vi "move manipulator abs xy.vi"(5 "blocking?":bool=TRUE, 7 "which manipulator":T1(ring), 8 "error in (no error)":errorcluster, 9 "transform cluster + actuator":T2, 10 "positions":T3, 11 "location (steps)":dbl[](array[numeric])) -> (0 "error out":errorcluster)   [LabVIEW 2015]
uses:
  pipette cleaning/pressure box/cleaning_soft/controls/actuator_type.ctl
  pipette cleaning/pressure box/cleaning_soft/controls/actuator_cluster.ctl
  machine_vision/coordinate model vis/transform_properties_actuators.ctl
  machine_vision/controls/transform_cluster_actuator.ctl
panel:
  # "move manip top lvl"
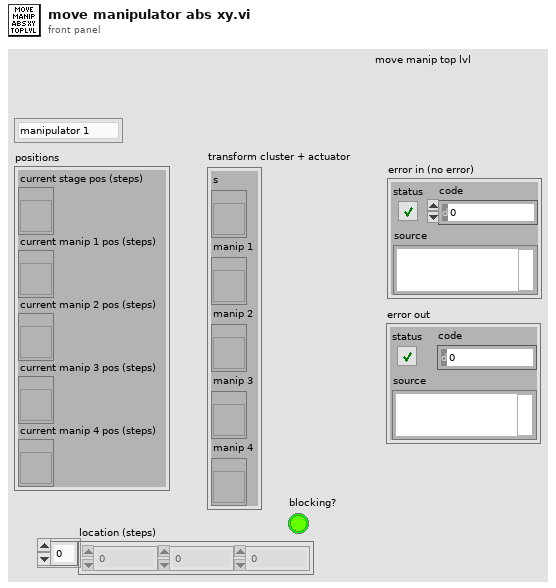
[diagram p1: front panel]
types:
  T1 = enum16{"manipulator 1", "manipulator 2", "manipulator 3", "manipulator 4"}
  T2 = typedef "transform_cluster_actuator.ctl" = cluster{"s":refnum<vi>, "manip 1":refnum<vi>, "manip 2":refnum<vi>, "manip 3":refnum<vi>, "manip 4":refnum<vi>}
  T3 = cluster{"current stage pos (steps)":refnum<vi>, "current manip 1 pos (steps)":refnum<vi>, "current manip 2 pos (steps)":refnum<vi>, "current manip 3 pos (steps)":refnum<vi>, "current manip 4 pos (steps)":refnum<vi>}
  T4 = typedef "transform_properties_actuators.ctl" = cluster{"theta (deg)":dbl, "X sc factor (px/step)":dbl, "Y sc factor (px/step)":dbl, "zero loc (x,y,z)":dbl[], "flip y?":bool, "flip x?":bool, "gamma (deg)":dbl, "flip z?":bool, "Z sc factor (px/step)":dbl, "actuator":T5, "safe space (steps)":i32[]}
  T5 = typedef "actuator_cluster.ctl" = cluster{"Actuator COM":refnum<visa-resource-name>, "Actuator type":T6}
  T6 = typedef "actuator_type.ctl" = enum16{"Scientifica", "Sutter", "Demo", "Off"}
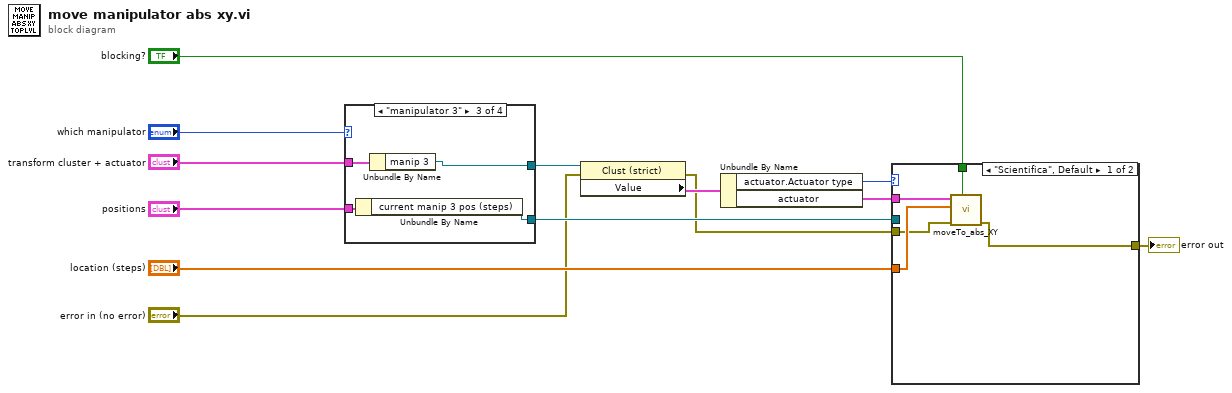
[diagram p0: block diagram]
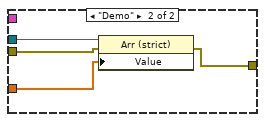
[diagram p2: hidden frame]
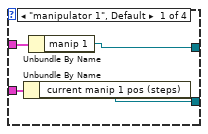
[diagram p3: hidden frame]
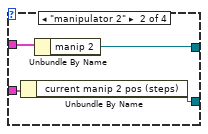
[diagram p4: hidden frame]
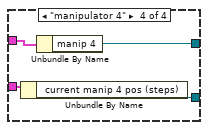
[diagram p5: hidden frame]
diagram:
  n1 = case shown="\"manipulator 3\"" "which manipulator" {
    tunnel: "transform cluster + actuator" -> [w17 w21 w25 w29]
    tunnel: [w16 w20 w24 w28] -> w9
    tunnel: "positions" -> [w15 w19 w23 w27]
    tunnel: [w14 w18 w22 w26] -> w5
    frame "manipulator 1", Default {
      n2 = Unbundle By Name(w15) -> ("current manip 1 pos (steps)"=w14:refnum<vi>)
      n3 = Unbundle By Name(w17) -> ("manip 1"=w16:refnum<vi>)
    }
    frame "manipulator 2" {
      n4 = Unbundle By Name(w19) -> ("current manip 2 pos (steps)"=w18:refnum<vi>)
      n5 = Unbundle By Name(w21) -> ("manip 2"=w20:refnum<vi>)
    }
    frame "manipulator 3" {
      n6 = Unbundle By Name(w23) -> ("current manip 3 pos (steps)"=w22:refnum<vi>)
      n7 = Unbundle By Name(w25) -> ("manip 3"=w24:refnum<vi>)
    }
    frame "manipulator 4" {
      n8 = Unbundle By Name(w27) -> ("current manip 4 pos (steps)"=w26:refnum<vi>)
      n9 = Unbundle By Name(w29) -> ("manip 4"=w28:refnum<vi>)
    }
  }
  n10 = property class="Clust (strict)"(reference=w9, error in="error in (no error)") -> (error out=w2:errorcluster, "Value"=w10:T4)  [unwired: 1 out]
  n11 = Unbundle By Name(w10) -> ("actuator.Actuator type"=w8:T6, "actuator"=w11:T5)
  n12 = case shown="\"Scientifica\", Default" w8 {
    tunnel: w11 -> [w34 _]
    tunnel: "blocking?" -> [w33 _]
    tunnel: w5 -> [_ w38]
    tunnel: "location (steps)" -> [w32 w37]
    tunnel: w2 -> [w31 w36]
    tunnel: [w30 w35] -> w1
    frame "Scientifica", Default {
      n13 = call "moveTo_abs_XY.vi"("blocking?"=w33, "error in"=w31, "XY location (steps)"=w32, "Actuator cluster in"=w34) -> ("error out"=w30:errorcluster)  [unwired: 6 in, 1 out]
    }
    frame "Demo" {
      n14 = property class="Arr (strict)"(reference=w38, error in=w36, "Value"=w37) -> (error out=w35:errorcluster)  [unwired: 1 out]
    }
  }
  "error out" <- w1
